vi "motortestMeng4.vi"() -> ()   [LabVIEW 2014]
doc: "Shows how to perform a relative motor move."
uses:
  <vilib>/Utility/inputDevices.llb/joystickAcquire.vi
  <vilib>/Utility/inputDevices.llb/closeJoystick.vi
panel:
  out "axis info":T1
  out "button info":T2
  in  "Motor":u16(ring) items=["X", "Y"]
  in  "MG17Motor":refnum<k7>(container)
  in  "Stop":bool
  in  "Home":bool
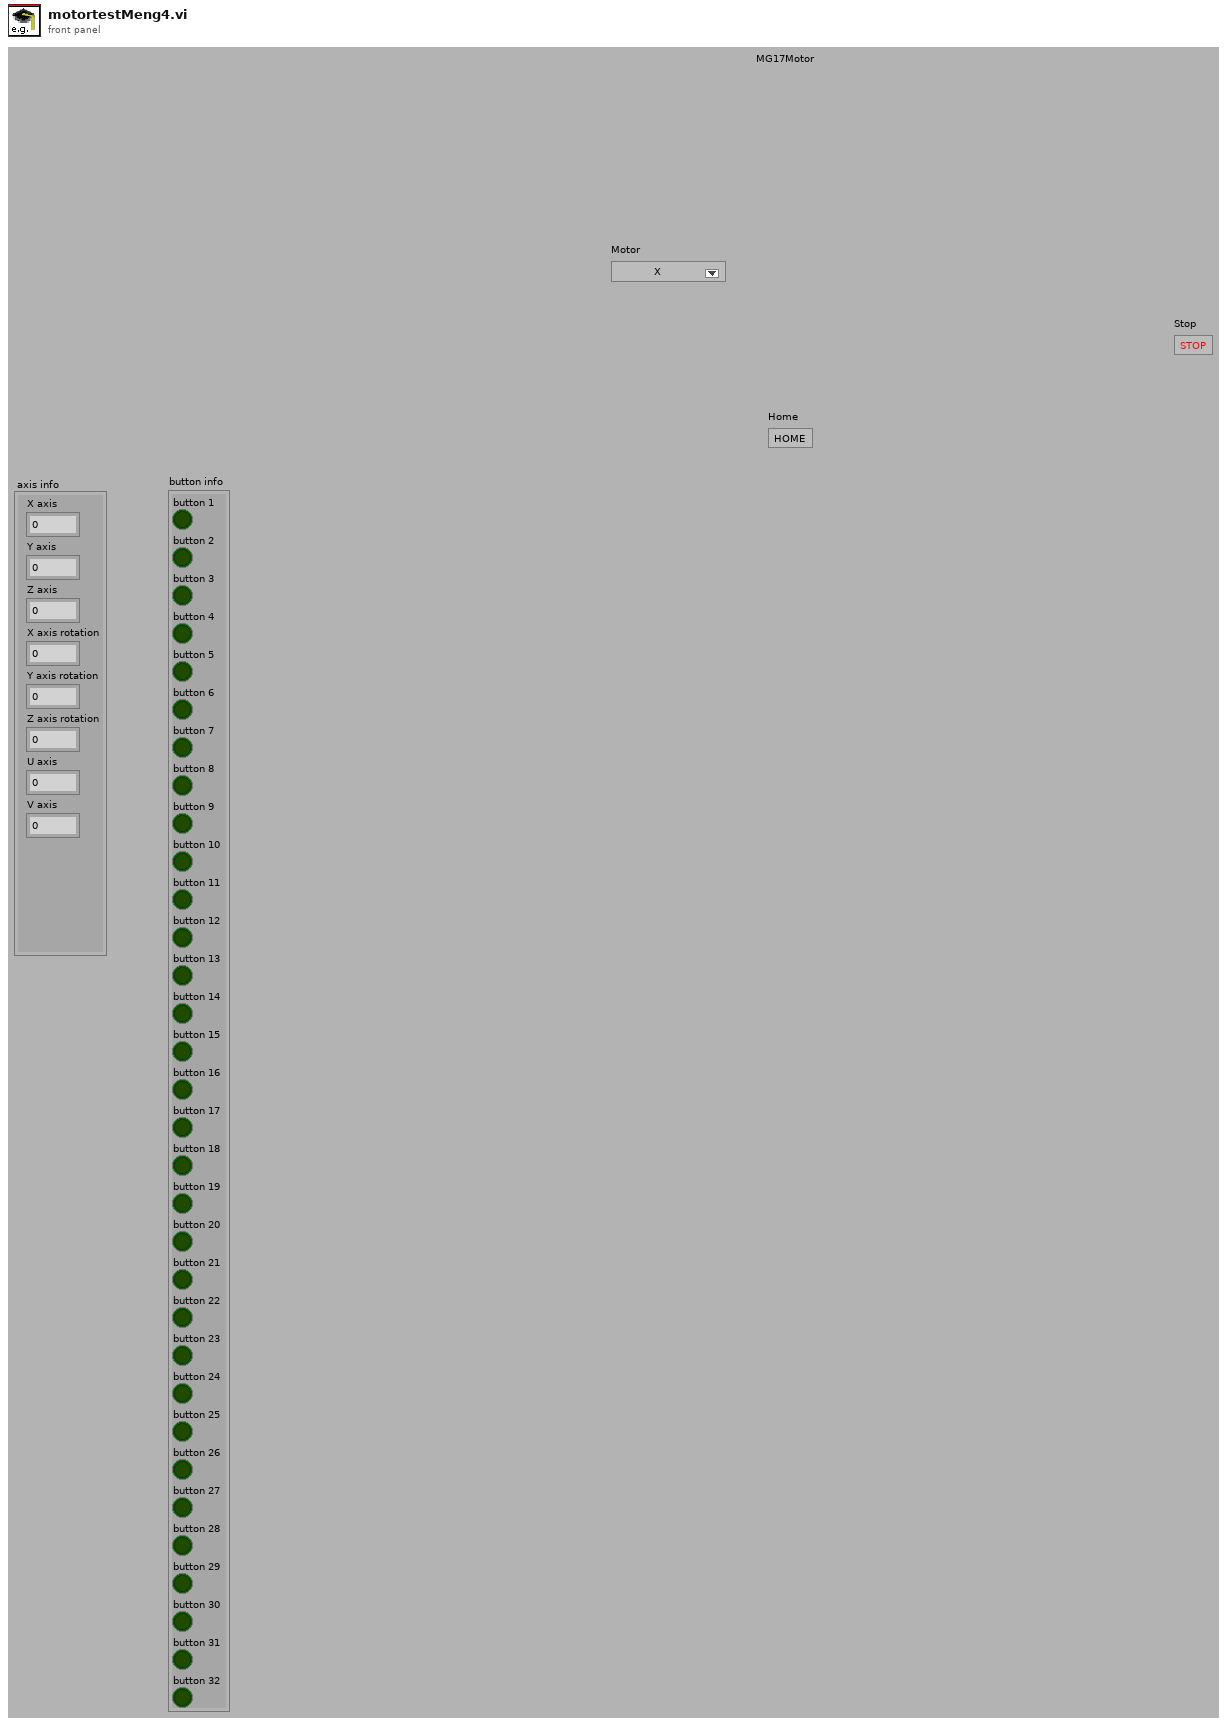
[diagram p1: front panel]
types:
  T1 = cluster{"X axis":i32, "Y axis":i32, "Z axis":i32, "X axis rotation":i32, "Y axis rotation":i32, "Z axis rotation":i32, "U axis":i32, "V axis":i32}
  T2 = cluster{"button 1":bool, "button 2":bool, "button 3":bool, "button 4":bool, "button 5":bool, "button 6":bool, "button 7":bool, "button 8":bool, "button 9":bool, "button 10":bool, "button 11":bool, "button 12":bool, "button 13":bool, "button 14":bool, "button 15":bool, "button 16":bool, "button 17":bool, "button 18":bool, "button 19":bool, "button 20":bool, "button 21":bool, "button 22":bool, "button 23":bool, "button 24":bool, "button 25":bool, "button 26":bool, "button 27":bool, "button 28":bool, "button 29":bool, "button 30":bool, "button 31":bool, "button 32":bool}
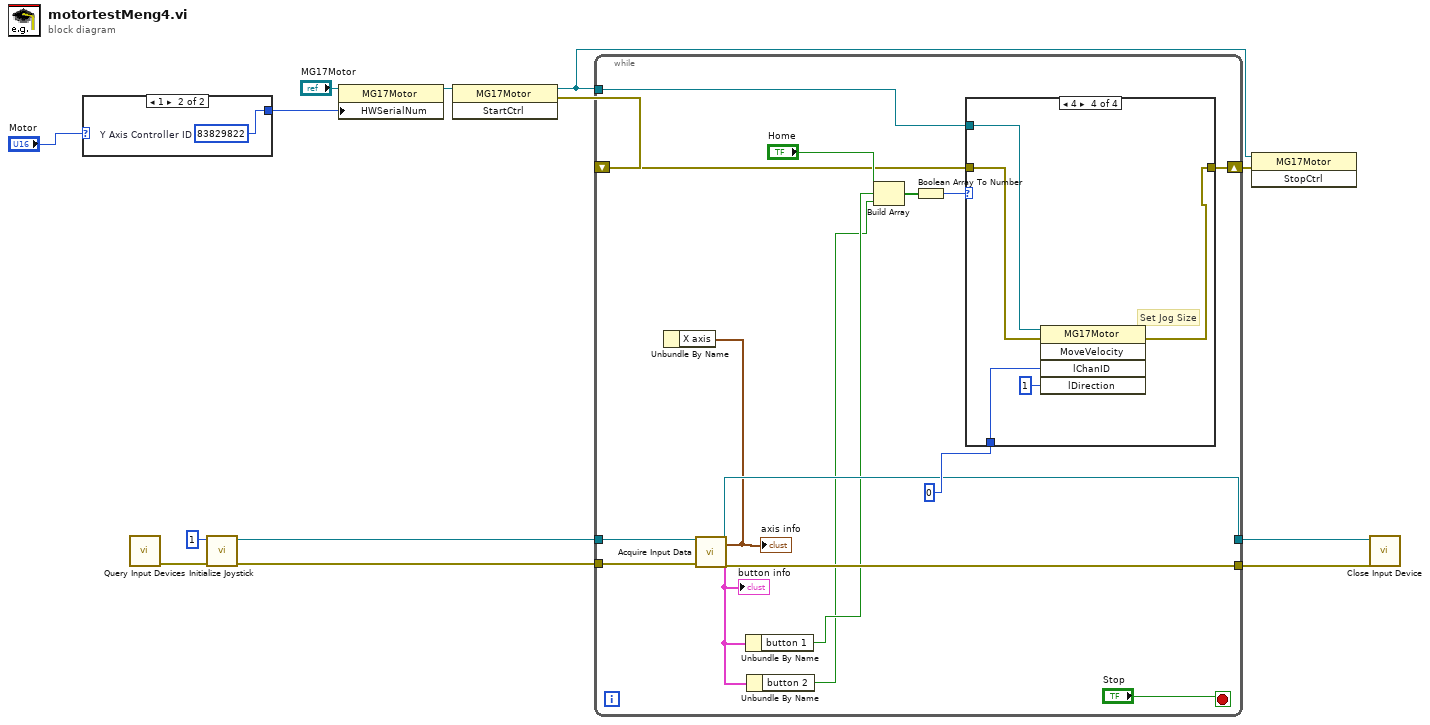
[diagram p0: block diagram]
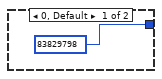
[diagram p2: hidden frame]
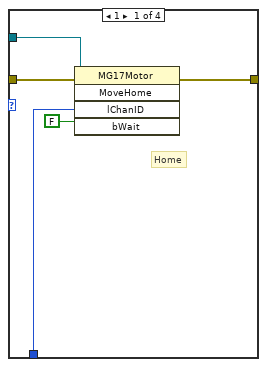
[diagram p3: hidden frame]
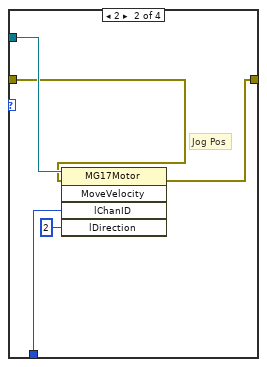
[diagram p4: hidden frame]
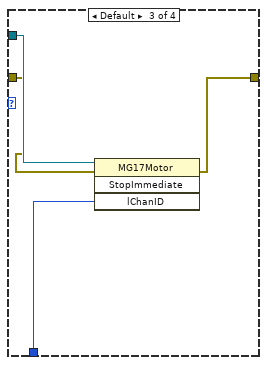
[diagram p5: hidden frame]
diagram:
  n1 = case shown="1" "Motor" {
    tunnel: [83829798 ("lChanID") w15] -> w10
    frame 0, Default {
    }
    frame 1 {
      w15 = 83829822  # Y Axis Controller ID
    }
  }
  n2 = call <vilib>:"Query Input Devices.vi"() -> ("error out"=w5:errorcluster)  [unwired: 8 in, 3 out]
  n3 = call <vilib>:"Initialize Joystick.vi"("error in (no error)"=w5, "device index"=1) -> ("error out"=w3:errorcluster, "device ID"=w4:refnum<k1>)  [unwired: 8 in]
  n4 = property class="MG17Motor"(reference="MG17Motor", "HWSerialNum"=w10) -> (reference out=w8:refnum<k7>)  [unwired: 1 in, 1 out]
  n5 = invoke class="MG17Motor" method="StartCtrl"(reference=w8) -> (reference out=w13:refnum<k7>, error out=w12:errorcluster)  [unwired: 2 in, 1 out]
  n6 = while {
    shift-left: w12 -> [w28]
    shift-right: [w29] -> w11
    tunnel: w13 -> [w20]
    tunnel: w4 -> [w24]
    tunnel: w3 -> [w23]
    tunnel: [w22] -> w2
    tunnel: [w21] -> w1
    stop <- "Stop" stop-if-true
    n7 = call-poly <vilib>:"Acquire Input Data.vi"("device ID"=w24, "error in (no error)"=w23) -> ("device ID 2"=w22:refnum<k1>, "axis info"=w16:T1, "button info"=w19:T2, "error out"=w21:errorcluster)  [unwired: 13 in, 1 out]
    "axis info" <- w16
    "button info" <- w19
    n8 = Unbundle By Name(w16) -> ()  [unwired: 1 out]
    n9 = Unbundle By Name(w19) -> ("button 1"=w18:bool)
    n10 = Unbundle By Name(w19) -> ("button 2"=w17:bool)
    n11 = Build Array("Home", w18, w17) -> (w25:bool[])
    n12 = Boolean Array To Number(Boolean array=w25) -> (number=w26:u32)
    n13 = case shown="4" w26 {
      tunnel: w20 -> [w36 w41 w45 w50]
      tunnel: 0 ("lChanID") -> [w35 w40 w42 w47]
      tunnel: [w34 w39 w44 w48] -> w29
      tunnel: w28 -> [w33 w38 w43 w49]
      frame 1 {
        # "Home"
        n14 = invoke class="MG17Motor" method="MoveHome"(reference=w36, error in=w33, "lChanID"=w35, "bWait"=FALSE) -> (error out=w34:errorcluster)  [unwired: 1 in, 4 out]
      }
      frame 2 {
        # "Jog Pos"
        n15 = invoke class="MG17Motor" method="MoveVelocity"(reference=w41, error in=w38, "lChanID"=w40, "lDirection"=2) -> (error out=w39:errorcluster)  [unwired: 1 in, 4 out]
      }
      frame Default {
        n16 = invoke class="MG17Motor" method="StopImmediate"(reference=w45, error in=w43, "lChanID"=w42) -> (error out=w44:errorcluster)  [unwired: 1 in, 3 out]
      }
      frame 4 {
        # "Set Jog Size"
        n17 = invoke class="MG17Motor" method="MoveVelocity"(reference=w50, error in=w49, "lChanID"=w47, "lDirection"=1) -> (error out=w48:errorcluster)  [unwired: 1 in, 4 out]
      }
    }
  }
  n18 = invoke class="MG17Motor" method="StopCtrl"(reference=w13, error in=w11) -> ()  [unwired: 1 in, 3 out]
  n19 = call-poly <vilib>:"Close Input Device.vi"("error in (no error)"=w1, "device ID"=w2) -> ()  [unwired: 8 in, 1 out]
